vi "ComunicacaoMedicao.vi"(8 "error in":errorcluster, 9 "Bool":bool[](array[boolean]), 10 "Palavra escrita":u16, 11 "Operação":T1(ring)) -> (0 "error out":errorcluster, 2 "BooleanLidos":bool[](array[boolean]), 3 "Valor":u16)   [LabVIEW 2019]
uses:
  TelaConfig/Configuracao.Variaveis.vi
  VariaveisMedicao.vi
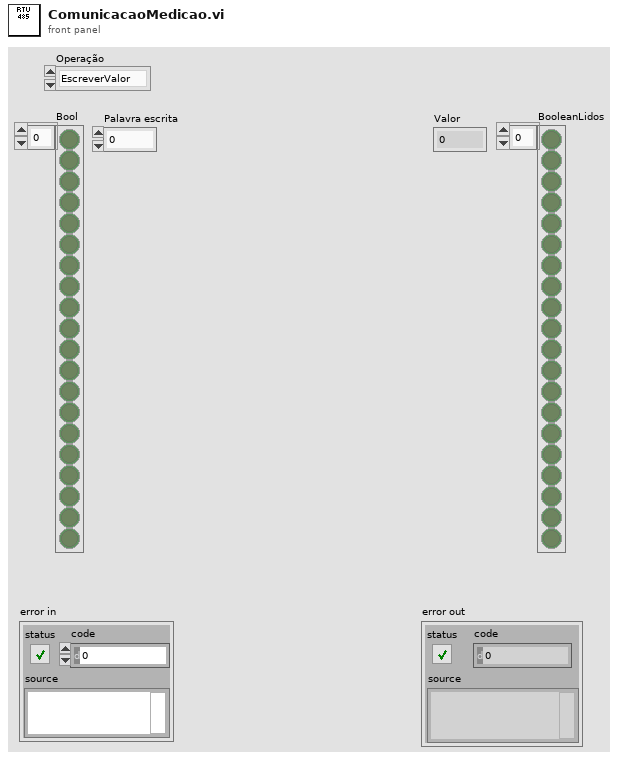
[diagram p1: front panel]
types:
  T1 = enum16{"EscreverValor", "LerValor", "EscreverBool", "LerBool", "OndaContinua", "IniciarRotação", "StatusInversor", "FinalizarRotacao"}
  T2 = enum16{"None", "Read Input Registers VI", "Read Discrete Inputs VI", "Read Holding Registers VI", "Read Coils VI", "Write Multiple Holding Registers", "Write Multiple Input Registers ", "Write Single Holding Registers"}
  T3 = cluster{"Operacao":enum16{"None", "Read Input Registers VI", "Read Discrete Inputs VI", "Read Holding Registers VI", "Read Coils VI", "Write Multiple Holding Registers", "Write Multiple Input Registers ", "Write Single Holding Registers"}, "Endereco":u16, "Número de palavras":u16, "Palavras":u16[], "Palavra escrita":u16}
  T4 = cluster{"Memoria":string, "TabelaPosicoesMemoria":string[][], "Status":bool[]}[]
  T5 = cluster{"Memoria":string, "TabelaPosicoesMemoria":string[][], "Status":bool[]}
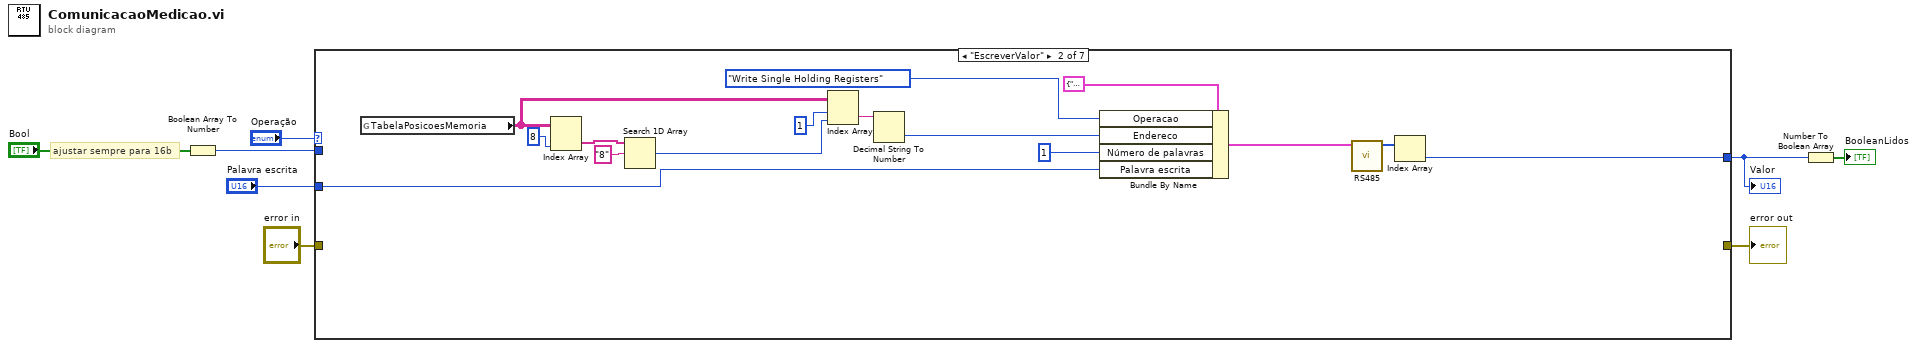
[diagram p0: block diagram]
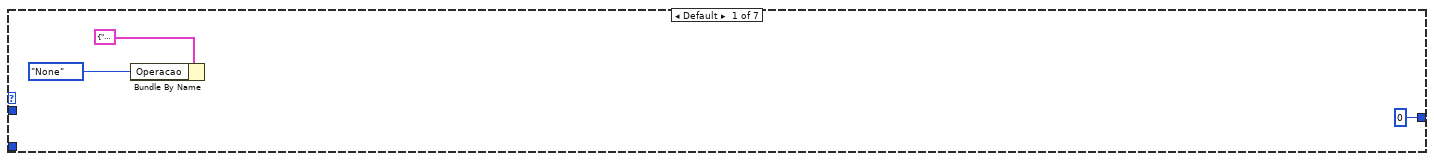
[diagram p2: hidden frame]
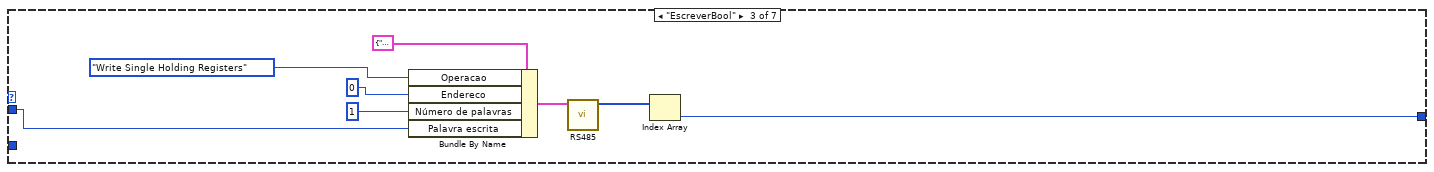
[diagram p3: hidden frame]
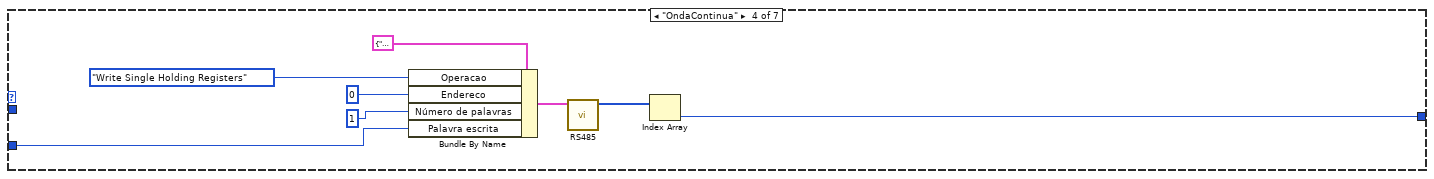
[diagram p4: hidden frame]
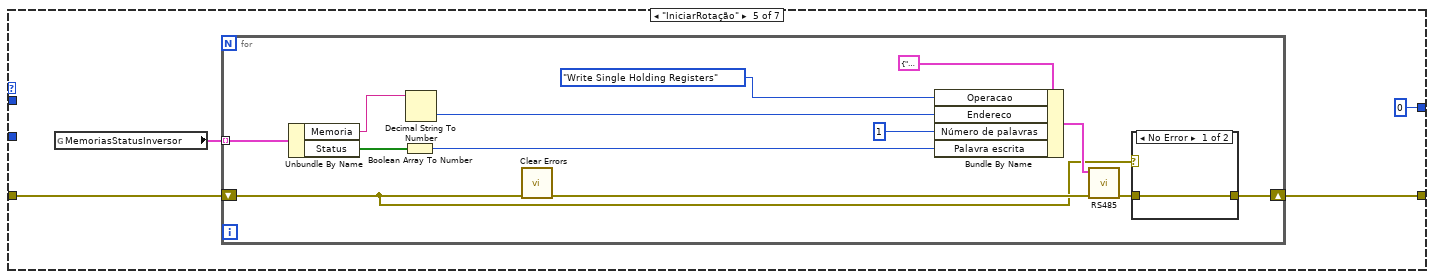
[diagram p5: hidden frame]
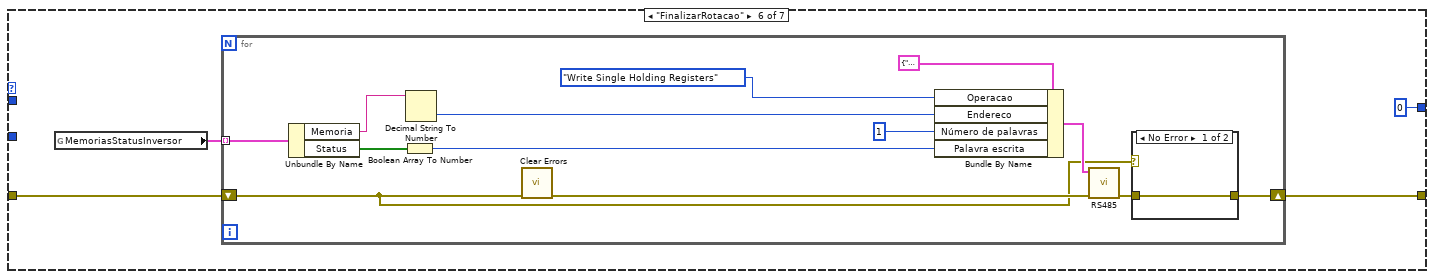
[diagram p7: hidden frame]
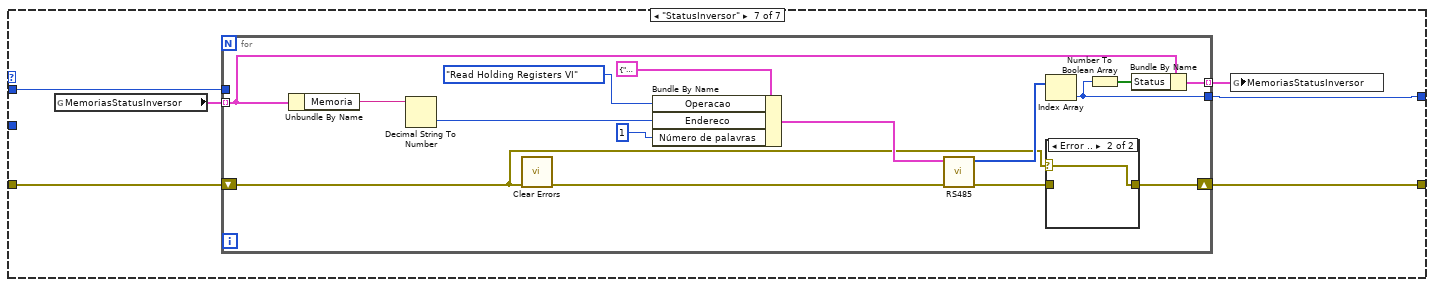
[diagram p9: hidden frame]
diagram:
  # "ajustar sempre para 16b"
  n1 = Boolean Array To Number(Boolean array="Bool") -> (number=w4:u32)
  n2 = case shown="\"EscreverValor\"" "Operação" {
    tunnel: "Palavra escrita" -> [_ w23 _ w35 _ _ _]
    tunnel: w4 -> [_ _ w30 _ _ _ w85]
    tunnel: [u16 0 ("register") w20 w27 w36 u16 0 ("register") u16 0 ("register") w86] -> w3
    tunnel: "error in" -> [_ _ _ _ w44 w63 w82]
    tunnel: [_ _ _ _ w43 w62 w81] -> w1
    frame Default {
      n3 = Bundle By Name(cluster=T3 {"Operacao"=enum."None", "Endereco"=0, "Número de palavras"=0, "Palavras"=[], "Palavra escrita"=0} ("ModbusIn"), "Operacao"=T2."None") -> ()  [unwired: 1 out]
    }
    frame "EscreverValor" {
      n4 = global read "Configuracao.Variaveis.vi" "TabelaPosicoesMemoria"() -> (w16:string[][])
      n5 = Index Array(array=w16, index (col)=8 ("disabled index (col)")) -> (element=w18:string[])  [unwired: 1 in]
      n6 = Search 1D Array(1D array=w18, element="8") -> (index of element=w15:i32)  [unwired: 1 in]
      n7 = Index Array(array=w16, index (row)=1 ("disabled index (row)"), index (col)=w15) -> (element=w13:string)
      n8 = Decimal String To Number(string=w13) -> (number=w12:i32)  [unwired: 2 in, 1 out]
      n9 = Bundle By Name(cluster=T3 {"Operacao"=enum."None", "Endereco"=0, "Número de palavras"=0, "Palavras"=[], "Palavra escrita"=0} ("ModbusIn"), "Operacao"=T2."Write Single Holding Registers", "Endereco"=w12, "Número de palavras"=u16 1, "Palavra escrita"=w23) -> (w21:T3)
      n10 = call "RS485.vi"("ModbusIn"=w21) -> ("ValoresLidos"=w22:u16[])  [unwired: 8 in, 1 out]
      n11 = Index Array(array=w22) -> (element=w20:u16)  [unwired: 1 in]
    }
    frame "EscreverBool" {
      n12 = Bundle By Name(cluster=T3 {"Operacao"=enum."None", "Endereco"=0, "Número de palavras"=0, "Palavras"=[], "Palavra escrita"=0} ("ModbusIn"), "Operacao"=T2."Write Single Holding Registers", "Endereco"=u16 0, "Número de palavras"=u16 1, "Palavra escrita"=w30) -> (w28:T3)
      n13 = call "RS485.vi"("ModbusIn"=w28) -> ("ValoresLidos"=w29:u16[])  [unwired: 8 in, 1 out]
      n14 = Index Array(array=w29) -> (element=w27:u16)  [unwired: 1 in]
    }
    frame "OndaContinua" {
      n15 = Bundle By Name(cluster=T3 {"Operacao"=enum."None", "Endereco"=0, "Número de palavras"=0, "Palavras"=[], "Palavra escrita"=0} ("ModbusIn"), "Operacao"=T2."Write Single Holding Registers", "Endereco"=u16 0, "Número de palavras"=u16 1, "Palavra escrita"=w35) -> (w37:T3)
      n16 = call "RS485.vi"("ModbusIn"=w37) -> ("ValoresLidos"=w38:u16[])  [unwired: 8 in, 1 out]
      n17 = Index Array(array=w38) -> (element=w36:u16)  [unwired: 1 in]
    }
    frame "IniciarRotação" {
      n18 = global read "VariaveisMedicao.vi" "MemoriasStatusInversor"() -> (w46:T4)
      n19 = for {
        tunnel: w46 -> [w55] mode=indexing
        shift-right: [w48] -> w43
        shift-left: w44 -> [w49]
        n20 = Unbundle By Name(w55) -> ("Memoria"=w54:string, "Status"=w52:bool[])
        n21 = Boolean Array To Number(Boolean array=w52) -> (number=w51:u32)
        n22 = Decimal String To Number(string=w54) -> (number=w53:i32)  [unwired: 2 in, 1 out]
        n23 = call <vilib>:"Clear Errors.vi"("error in (no error)"=w49) -> ("error out"=w50:errorcluster)  [unwired: 5 in, 1 out]
        n24 = Bundle By Name(cluster=T3 {"Operacao"=enum."None", "Endereco"=0, "Número de palavras"=0, "Palavras"=[], "Palavra escrita"=0} ("ModbusIn"), "Operacao"=T2."Write Single Holding Registers", "Endereco"=w53, "Número de palavras"=u16 1, "Palavra escrita"=w51) -> (w56:T3)
        n25 = call "RS485.vi"("ModbusIn"=w56, "error in"=w50) -> ("error out"=w47:errorcluster)  [unwired: 7 in, 1 out]
        n26 = case shown="No Error" w49 {
          selector: w49 -> [_ w61]
          tunnel: [w60 w61] -> w48
          tunnel: w47 -> [w60 _]
          frame No Error {
          }
          frame Error {
          }
        }
      }
    }
    frame "FinalizarRotacao" {
      n27 = global read "VariaveisMedicao.vi" "MemoriasStatusInversor"() -> (w65:T4)
      n28 = for {
        tunnel: w65 -> [w74] mode=indexing
        shift-right: [w67] -> w62
        shift-left: w63 -> [w68]
        n29 = Unbundle By Name(w74) -> ("Memoria"=w73:string, "Status"=w71:bool[])
        n30 = Boolean Array To Number(Boolean array=w71) -> (number=w70:u32)
        n31 = Decimal String To Number(string=w73) -> (number=w72:i32)  [unwired: 2 in, 1 out]
        n32 = call <vilib>:"Clear Errors.vi"("error in (no error)"=w68) -> ("error out"=w69:errorcluster)  [unwired: 5 in, 1 out]
        n33 = Bundle By Name(cluster=T3 {"Operacao"=enum."None", "Endereco"=0, "Número de palavras"=0, "Palavras"=[], "Palavra escrita"=0} ("ModbusIn"), "Operacao"=T2."Write Single Holding Registers", "Endereco"=w72, "Número de palavras"=u16 1, "Palavra escrita"=w70) -> (w75:T3)
        n34 = call "RS485.vi"("ModbusIn"=w75, "error in"=w69) -> ("error out"=w66:errorcluster)  [unwired: 7 in, 1 out]
        n35 = case shown="No Error" w68 {
          selector: w68 -> [_ w80]
          tunnel: [w79 w80] -> w67
          tunnel: w66 -> [w79 _]
          frame No Error {
          }
          frame Error {
          }
        }
      }
    }
    frame "StatusInversor" {
      n36 = global read "VariaveisMedicao.vi" "MemoriasStatusInversor"() -> (w84:T4)
      n37 = for {
        tunnel: [w96] -> w86
        tunnel: w85 -> [_]
        tunnel: w84 -> [w95] mode=indexing
        tunnel: [w93] -> w83 mode=indexing
        shift-right: [w88] -> w81
        shift-left: w82 -> [w89]
        n38 = Unbundle By Name(w95) -> ("Memoria"=w97:string)
        n39 = Decimal String To Number(string=w97) -> (number=w92:i32)  [unwired: 2 in, 1 out]
        n40 = call <vilib>:"Clear Errors.vi"("error in (no error)"=w89) -> ("error out"=w90:errorcluster)  [unwired: 5 in, 1 out]
        n41 = Bundle By Name(cluster=T3 {"Operacao"=enum."None", "Endereco"=0, "Número de palavras"=0, "Palavras"=[], "Palavra escrita"=0} ("ModbusIn"), "Operacao"=T2."Read Holding Registers VI", "Endereco"=w92, "Número de palavras"=u16 1) -> (w98:T3)
        n42 = call "RS485.vi"("ModbusIn"=w98, "error in"=w90) -> ("ValoresLidos"=w99:u16[], "error out"=w87:errorcluster)  [unwired: 7 in]
        n43 = Index Array(array=w99) -> (element=w96:u16)  [unwired: 1 in]
        n44 = case shown="Error .." w89 {
          selector: w89 -> [_ w103]
          tunnel: [w102 w103] -> w88
          tunnel: w87 -> [w102 _]
          frame No Error {
          }
          frame Error {
          }
        }
        n45 = Number To Boolean Array(number=w96) -> (Boolean array=w94:bool[])
        n46 = Bundle By Name(cluster=w95, "Status"=w94) -> (w93:T5)
      }
      n47 = global write "VariaveisMedicao.vi" "MemoriasStatusInversor"(w83) -> ()
    }
  }
  "Valor" <- w3
  "error out" <- w1
  n48 = Number To Boolean Array(number=w3) -> (Boolean array=→"BooleanLidos":bool[])
